vi "ForwardMotor.vi"(9 "Go":bool, 10 "stop":bool, 11 "Speed (km/h)":u16) -> ()   [LabVIEW 2019]
panel:
  out "error out":errorcluster
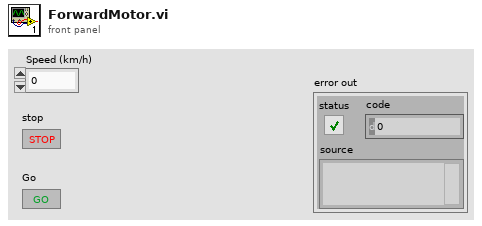
[diagram p1: front panel]
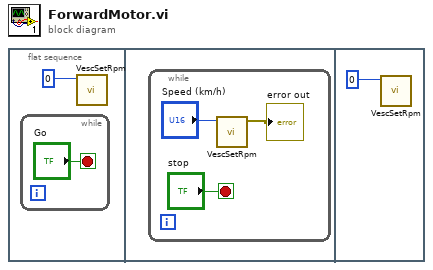
[diagram p0: block diagram]
diagram:
  n1 = flat-sequence {
    frame #0 {
      n2 = while {
        stop <- "Go" stop-if-true
      }
      n3 = call "VescSetRpm.vi"("Speed (rpm)"=0) -> ()  [unwired: 10 in, 1 out]
    }
    frame #1 {
      n4 = while {
        stop <- "stop" stop-if-true
        n5 = call "VescSetRpm.vi"("Speed (rpm)"="Speed (km/h)") -> ("error out"=→"error out":errorcluster)  [unwired: 10 in]
      }
    }
    frame #2 {
      n6 = call "VescSetRpm.vi"("Speed (rpm)"=0) -> ()  [unwired: 10 in, 1 out]
    }
  }
